vi "FGV_OBJ_test_button.vi"(4 "OBJ_test_button":refnum<vi>, 6 "operator_message":refnum<vi>, 7 "options":T1, 8 "error_in":errorcluster, 9 "scan_tooling":bool, 11 "input":variant) -> (0 "error_out":errorcluster, 1 "scan_tooling?":bool)   [LabVIEW 2020]
uses:
  FGV_OBJ_test_button.ctl
  _misc/AULocalize/SubVIs/Get Localized Phrase Compact Interface 0D.vi
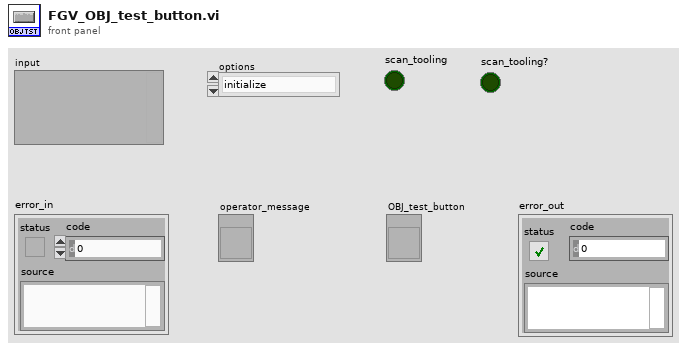
[diagram p1: front panel]
types:
  T1 = typedef "FGV_OBJ_test_button.ctl" = enum16{"initialize", "set_new_login", "set_message", "enable", "disable", "disable_gray", "translate", "set_scan_tooling", "get_scan_tooling"}
  T2 = enum8{"Enabled", "Disabled", "Disabled and Grayed Out"}
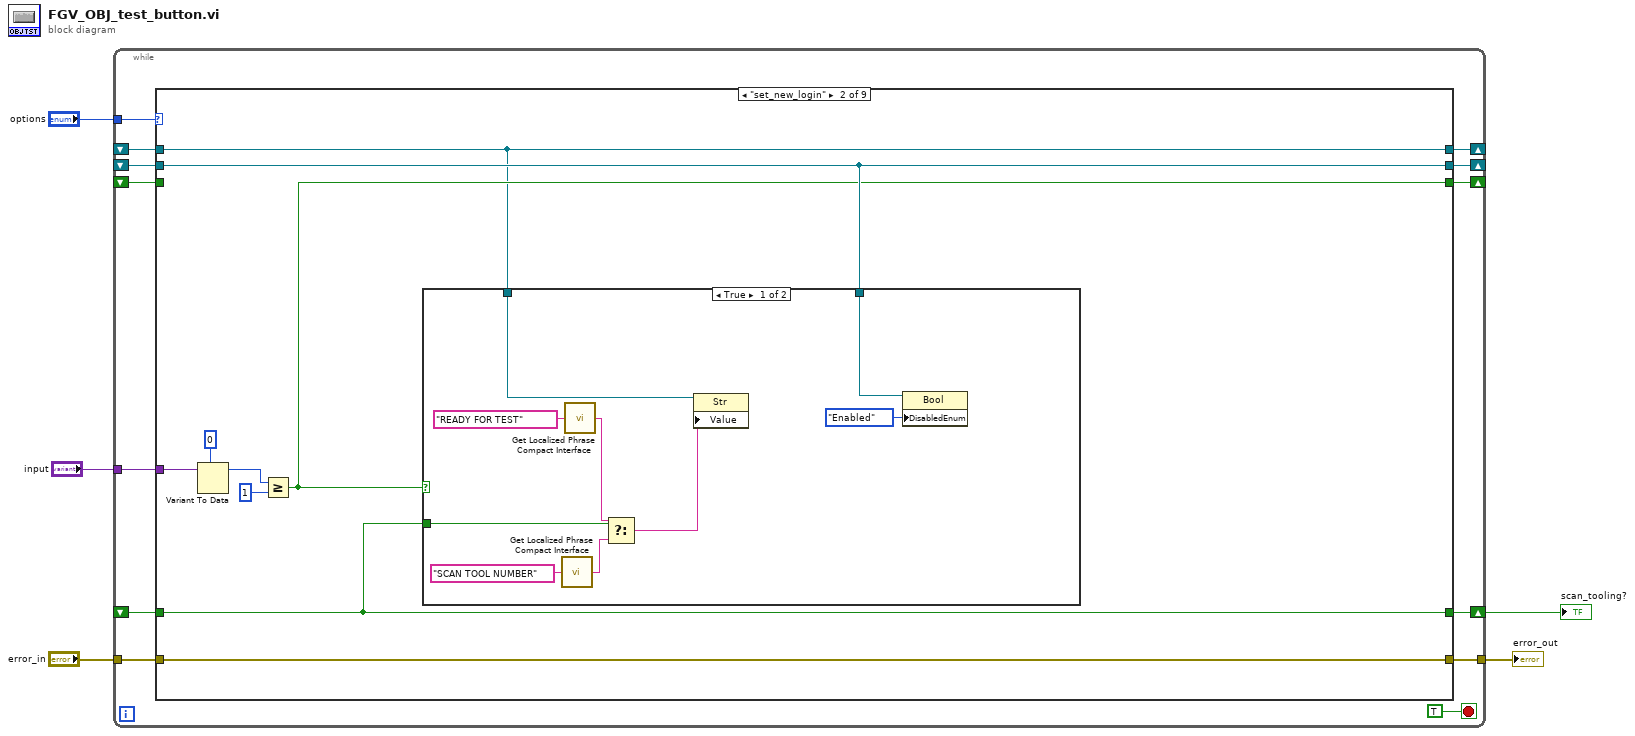
[diagram p0: block diagram]
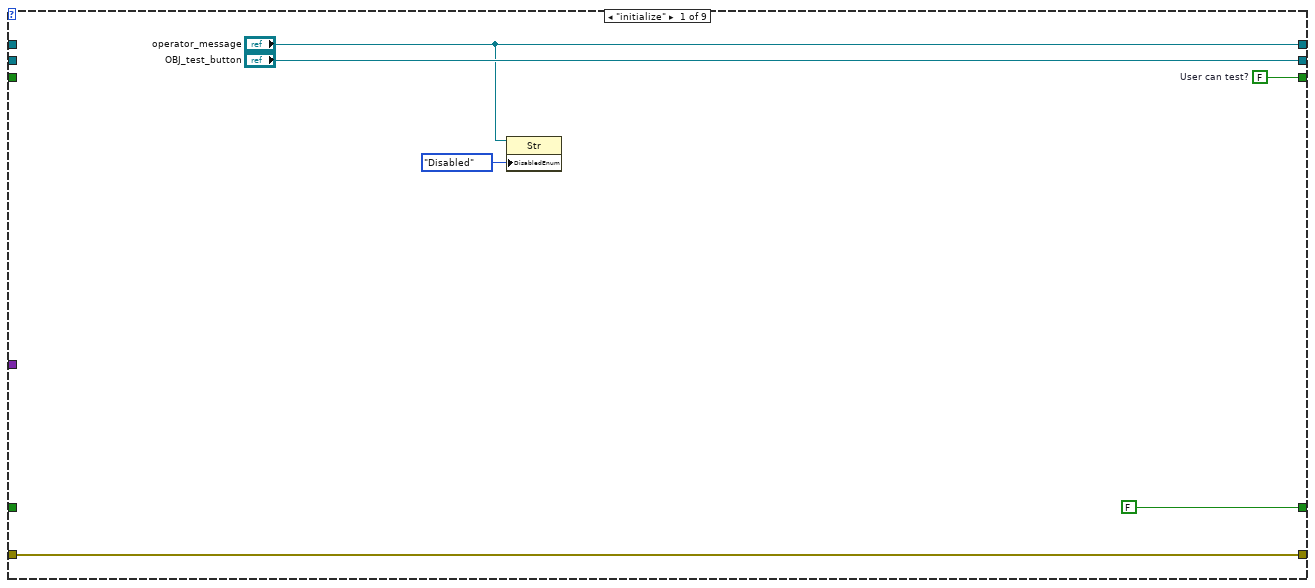
[diagram p2: hidden frame]
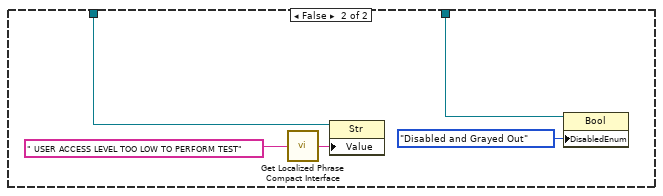
[diagram p3: hidden frame]
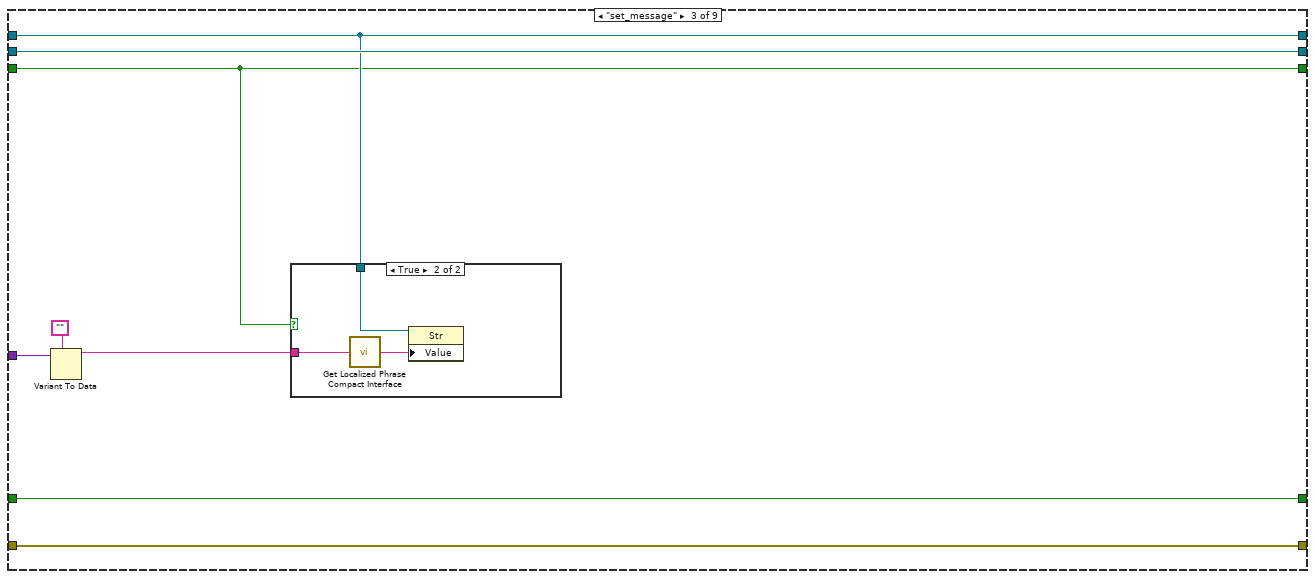
[diagram p4: hidden frame]
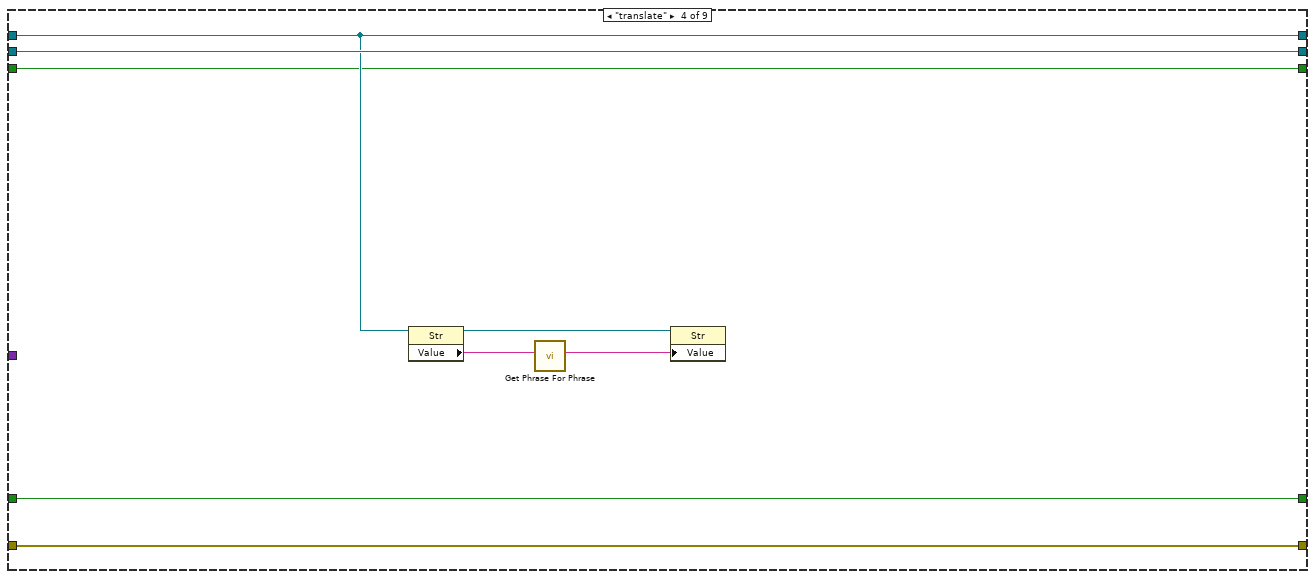
[diagram p6: hidden frame]
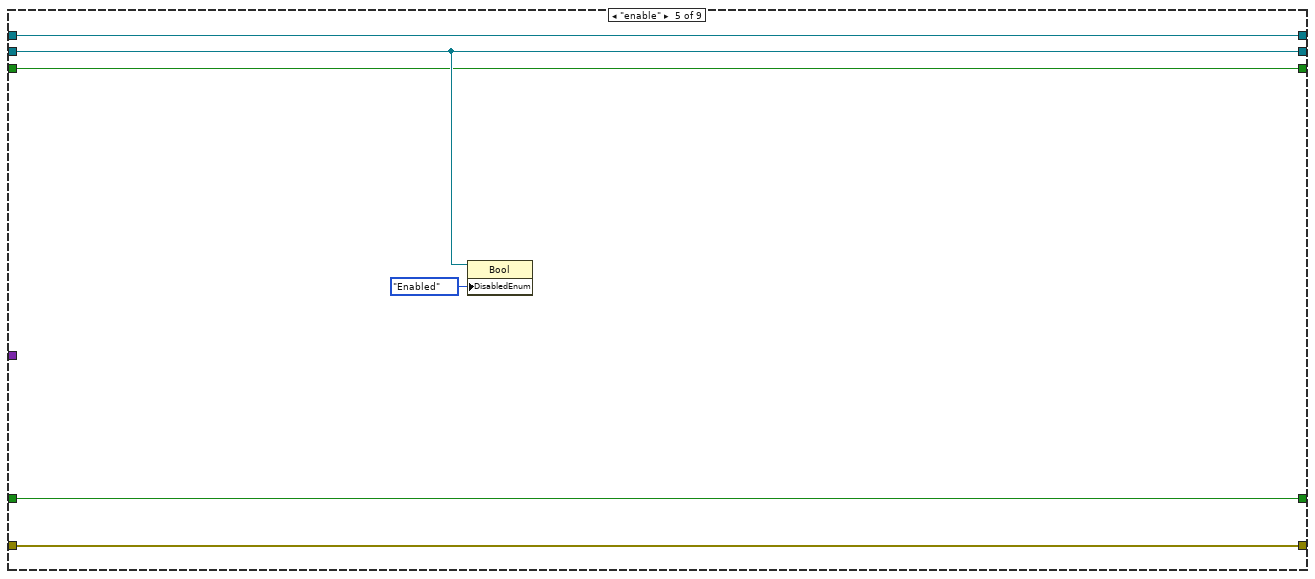
[diagram p7: hidden frame]
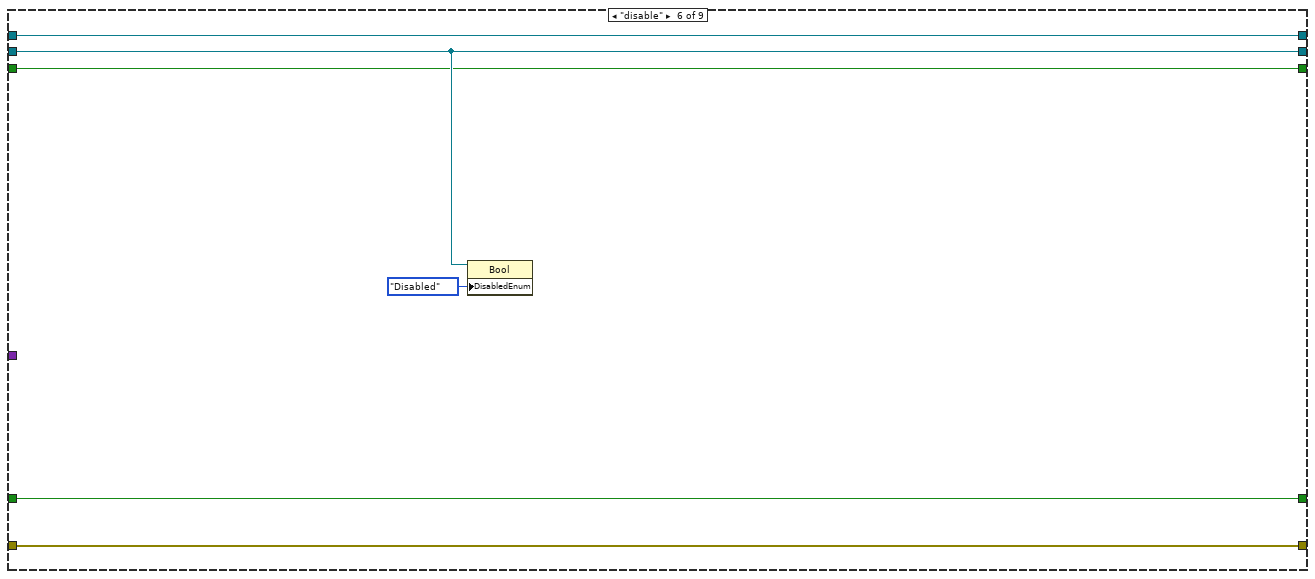
[diagram p8: hidden frame]
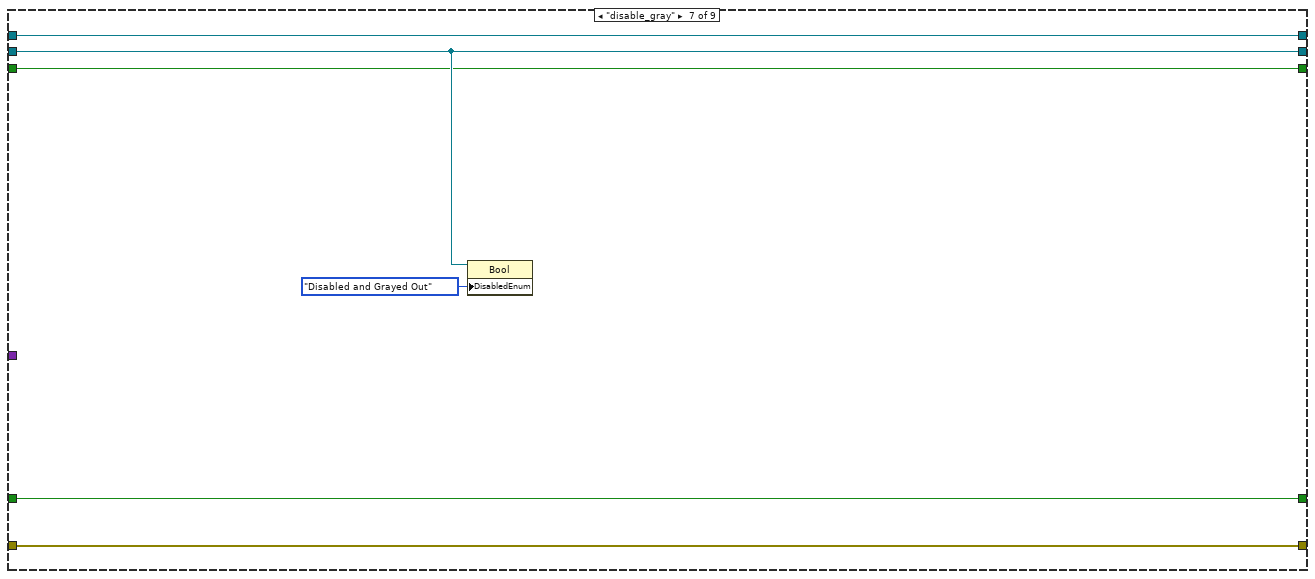
[diagram p9: hidden frame]
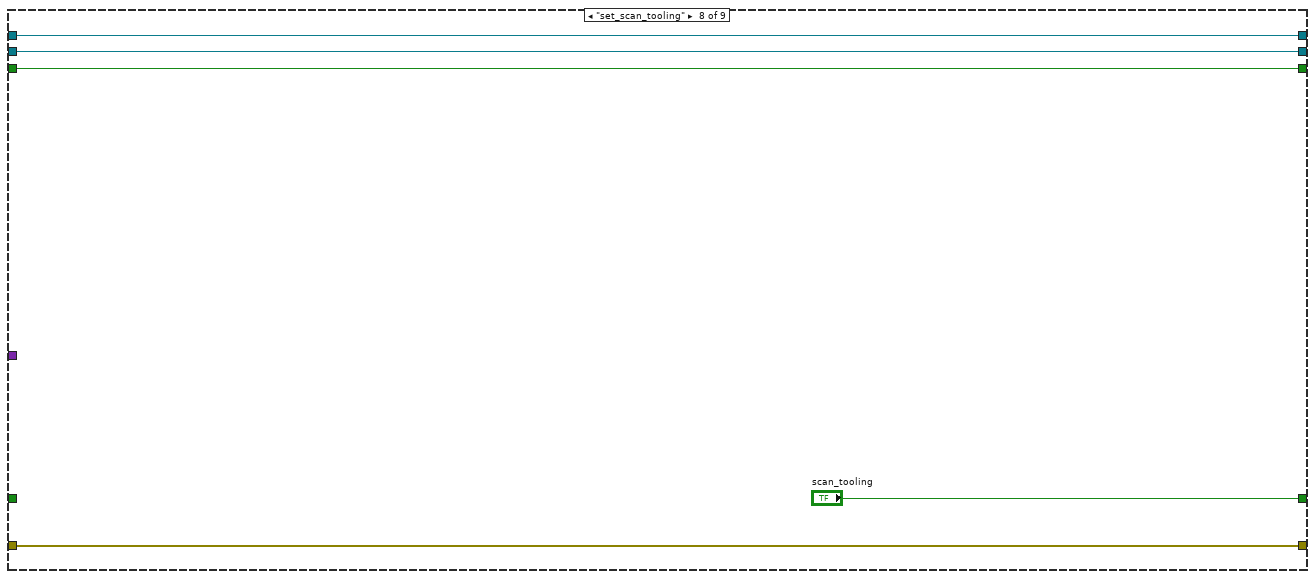
[diagram p10: hidden frame]
diagram:
  n1 = while {
    tunnel: "options" -> [w17]
    tunnel: [w16] -> w5
    tunnel: "error_in" -> [w15]
    tunnel: "input" -> [w14]
    shift-right: [w13] -> _
    shift-left: _ -> [w12]
    shift-right: [w11] -> _
    shift-left: _ -> [w10]
    shift-right: [w9] -> _
    shift-left: _ -> [w8]
    shift-right: [w7] -> w1
    shift-left: _ -> [w6]
    stop <- TRUE stop-if-true
    n2 = case shown="\"set_new_login\"" w17 {
      tunnel: [w24 w33 w55 w66 w72 w78 w84 w89 w94] -> w16
      tunnel: w15 -> [w24 w33 w55 w66 w72 w78 w84 w89 w94]
      tunnel: w14 -> [_ w31 w53 _ _ _ _ _ _]
      tunnel: ["OBJ_test_button" w32 w54 w65 w70 w76 w82 w88 w93] -> w13
      tunnel: w12 -> [_ w32 w54 w65 w70 w76 w82 w88 w93]
      tunnel: [w23 w27 w49 w63 w69 w75 w81 w87 w92] -> w11
      tunnel: w10 -> [_ _ w49 w63 w69 w75 w81 w87 w92]
      tunnel: ["operator_message" w26 w52 w64 w68 w74 w80 w86 w91] -> w9
      tunnel: w8 -> [_ w26 w52 w64 w68 w74 w80 w86 w91]
      tunnel: [FALSE w25 w48 w59 w67 w73 w79 "scan_tooling" w90] -> w7
      tunnel: w6 -> [_ w25 w48 w59 w67 w73 w79 _ w90]
      frame "initialize" {
        w23 = FALSE  # User can test?
        n3 = property class="Str"(reference="operator_message", "DisabledEnum"=T2."Disabled" ("Disabled")) -> ()  [unwired: 1 in, 2 out]
      }
      frame "set_new_login" {
        n4 = Variant To Data(type=0 ("y"), Variant=w31) -> (data=w28:i32)  [unwired: 1 in, 1 out]
        n5 = Greater Or Equal?(x=w28, y=1) -> (x >= y?=w27:bool)
        n6 = case shown="True" w27 {
          tunnel: w26 -> [w42 w45]
          tunnel: w32 -> [w41 w47]
          tunnel: w25 -> [w38 _]
          frame True {
            n7 = call-poly "Get Localized Phrase Compact Interface.vi"("Key"="SCAN TOOL NUMBER" ("String")) -> ("Translated Phrase"=w35:string)
            n8 = call-poly "Get Localized Phrase Compact Interface.vi"("Key"="READY FOR TEST" ("String")) -> ("Translated Phrase"=w37:string)
            n9 = Select(t=w37, s=w38, f=w35) -> (s? t:f=w34:string)
            n10 = property class="Str"(reference=w42, "Value"=w34) -> ()  [unwired: 1 in, 2 out]
            n11 = property class="Bool"(reference=w41, "DisabledEnum"=T2."Enabled" ("Disabled")) -> ()  [unwired: 1 in, 2 out]
          }
          frame False {
            n12 = call-poly "Get Localized Phrase Compact Interface.vi"("Key"=" USER ACCESS LEVEL TOO LOW TO PERFORM TEST" ("String")) -> ("Translated Phrase"=w43:string)
            n13 = property class="Str"(reference=w45, "Value"=w43) -> ()  [unwired: 1 in, 2 out]
            n14 = property class="Bool"(reference=w47, "DisabledEnum"=T2."Disabled and Grayed Out" ("Disabled")) -> ()  [unwired: 1 in, 2 out]
          }
        }
      }
      frame "set_message" {
        n15 = Variant To Data(type="", Variant=w53) -> (data=w50:string)  [unwired: 1 in, 1 out]
        n16 = case shown="True" w49 {
          tunnel: w52 -> [_ w58]
          tunnel: w50 -> [_ w57]
          frame False {
          }
          frame True {
            n17 = call-poly "Get Localized Phrase Compact Interface.vi"("Key"=w57) -> ("Translated Phrase"=w56:string)
            n18 = property class="Str"(reference=w58, "Value"=w56) -> ()  [unwired: 1 in, 2 out]
          }
        }
      }
      frame "translate" {
        n19 = property class="Str"(reference=w64) -> (reference out=w60:refnum<vi>, "Value"=w62:string)  [unwired: 1 in, 1 out]
        n20 = call "Get Phrase For Phrase.vi"("Phrase"=w62) -> ("Phrase"=w61:string)  [unwired: 9 in, 1 out]
        n21 = property class="Str"(reference=w60, "Value"=w61) -> ()  [unwired: 1 in, 2 out]
      }
      frame "enable" {
        n22 = property class="Bool"(reference=w70, "DisabledEnum"=T2."Enabled" ("Disabled")) -> ()  [unwired: 1 in, 2 out]
      }
      frame "disable" {
        n23 = property class="Bool"(reference=w76, "DisabledEnum"=T2."Disabled" ("Disabled")) -> ()  [unwired: 1 in, 2 out]
      }
      frame "disable_gray" {
        n24 = property class="Bool"(reference=w82, "DisabledEnum"=T2."Disabled and Grayed Out" ("Disabled")) -> ()  [unwired: 1 in, 2 out]
      }
      frame "set_scan_tooling" {
      }
      frame "get_scan_tooling" {
      }
    }
  }
  "error_out" <- w5
  "scan_tooling?" <- w1
